vi "Write Timestamp Options.vi"(10 "Timestamp Serialization":T1, 11 "Serializer.JSON in":refnum<class "Serializer.JSON.lvclass">) -> (3 "Serializer.JSON out":refnum<class "Serializer.JSON.lvclass">)   [LabVIEW 2019, in "OpenSerializer.JKI-JSON.lvlib" / "Serializer.JSON.lvclass"]
uses:
  Serializer.JSON.lvclass
  <vilib>/addons/_JKI.lib/Serialization/JSON/Library/Timestamp Options.ctl
  <vilib>/addons/_JKI.lib/Serialization/JSON/JKI JSON Serialization.lvlib
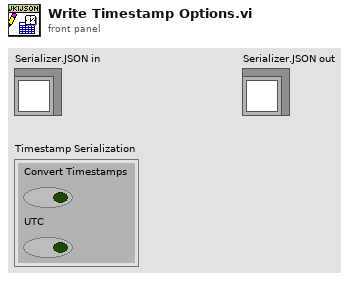
[diagram p1: front panel]
types:
  T1 = typedef "JKI JSON Serialization.lvlib/Timestamp Options.ctl" = cluster{"Convert Timestamps":bool, "UTC":bool}
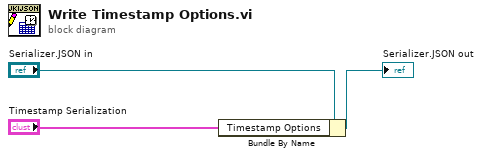
[diagram p0: block diagram]
diagram:
  n1 = Bundle By Name(cluster="Serializer.JSON in", "Timestamp Options"="Timestamp Serialization") -> (→"Serializer.JSON out":refnum<class "Serializer.JSON.lvclass">)
